vi "周围地雷个数.vi"(1 "索引":i32) -> (0 "数值":i32)   [LabVIEW 2017]
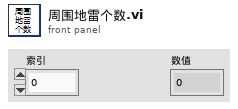
[diagram p1: front panel]
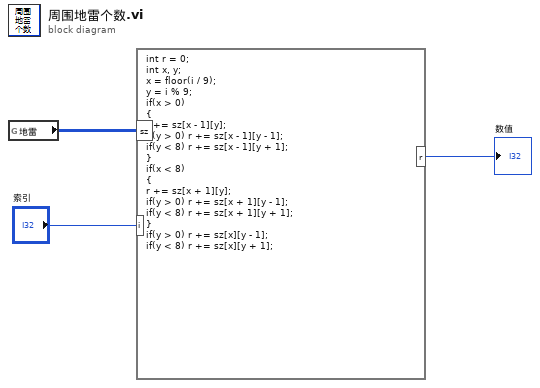
[diagram p0: block diagram]
diagram:
  n1 = global read "全局 地雷数组.vi" "地雷"() -> (w1:i16[][])
  n2 = formula code="int r = 0;\nint x, y;\nx = floor(i / 9);\ny = i % 9;\nif(x > 0)\n{\nr += sz[x - 1][y];\nif(y > 0) r += sz[x - 1][y - 1];\nif(y < 8) r += sz[x - 1][y + 1];\n}\nif(x < 8)\n{\nr += sz[x + 1][y];\nif(y > 0) r += sz[x + 1][y - 1];\nif(y < 8) r += sz[x + 1][y + 1];\n}\nif(y > 0) r += sz[x][y - 1];\nif(y < 8) r += sz[x][y + 1];"("sz"=w1, "i"="索引") -> ("r"=→"数值":i32)
